vi "Calculate Frame Size.vi"(11 "Parameters":T1[](array[typedef]) {"Byte Order" items=["Little Endian", "Big Endian"]; "Data Type" items=["Signed", "Unsigned", "IEEE Float"]}) -> (3 "Bytes":u8)   [LabVIEW 2015, in "Diagnostics Addon Shared.lvlib"]
uses:
  Types/Signal Parameters.ctl
  Diagnostics Addon Shared.lvlib
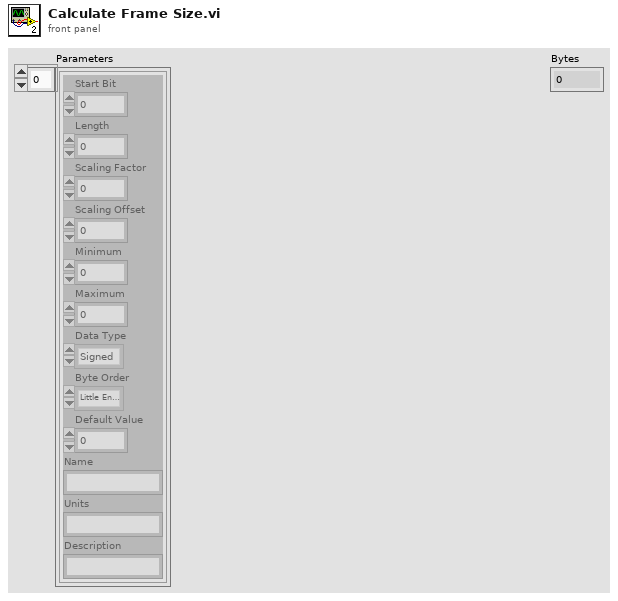
[diagram p1: front panel]
types:
  T1 = typedef "Diagnostics Addon Shared.lvlib/Signal Parameters.ctl" = cluster{"Start Bit":u8, "Length":u8, "Scaling Factor":dbl, "Scaling Offset":dbl, "Minimum":dbl, "Maximum":dbl, "Data Type":u32, "Byte Order":u32, "Default Value":dbl, "Name":string, "Units":string, "Description":string}
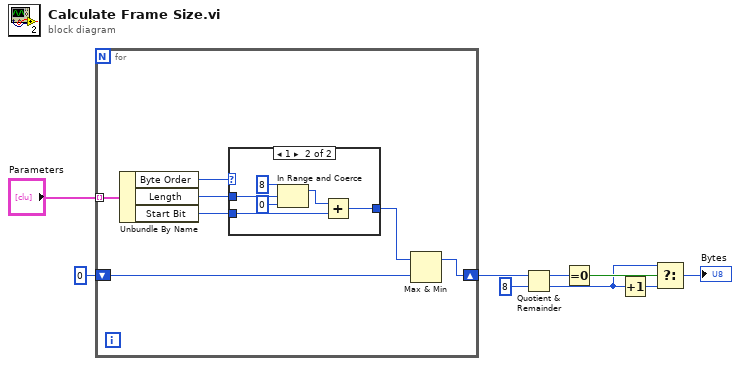
[diagram p0: block diagram]
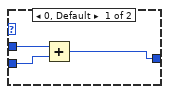
[diagram p2: hidden frame]
diagram:
  n1 = for {
    tunnel: "Parameters" -> [w16] mode=indexing
    shift-right: [w14] -> w7
    shift-left: u8 0 -> [w15]
    n2 = Unbundle By Name(w16) -> ("Byte Order"=w13:u32, "Length"=w12:u8, "Start Bit"=w11:u8)
    n3 = case shown="1" w13 {
      tunnel: w12 -> [w19 w24]
      tunnel: w11 -> [w18 w25]
      tunnel: [w17 w20] -> w10
      frame 0, Default {
        n4 = Add(x=w19, y=w18) -> (x+y=w17:u8)
      }
      frame 1 {
        n5 = In Range and Coerce(upper limit=u8 8, x=w24, lower limit=u8 0) -> (coerced(x)=w21:u8)  [unwired: 1 out]
        n6 = Add(x=w21, y=w25) -> (x+y=w20:u8)
      }
    }
    n7 = Max & Min(x=w10, y=w15) -> (max(x,y)=w14:u8)  [unwired: 1 out]
  }
  n8 = Quotient & Remainder(x=w7, y=u8 8) -> (x-y*floor(x/y)=w5:u8, floor(x/y)=w3:u8)
  n9 = Equal To 0?(x=w5) -> (x = 0?=w4:bool)
  n10 = Increment(x=w3) -> (x+1=w2:u8)
  n11 = Select(t=w3, s=w4, f=w2) -> (s? t:f=→"Bytes":u8)
